vi "Teardown.vi"(6 "Error":errorcluster, 7 "Actor":refnum<class "Actor.lvclass">, 11 "UnhandledMessages":refnum<class "Message.lvclass">[](array[class])) -> ()   [LabVIEW 2020, in "jettl.lvlib" / "Base.lvlib" / "Actor.lvclass"]
uses:
  Actor.lvclass
  Actor.lvclass/Actor.ctl
  Message/Message.lvclass
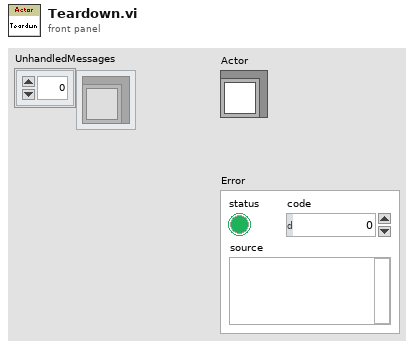
[diagram p1: front panel]
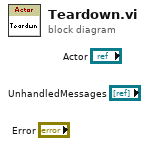
[diagram p0: block diagram]
diagram:
